vi "Launcher.vi"() -> ()   [LabVIEW 2022 SP3]
uses:
  Dynamic Load/Dynamic Load.lvclass
panel:
  in  "Dynamic Load.lvclass":refnum<class "Dynamic Load.lvclass">
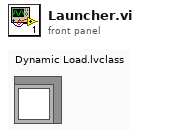
[diagram p1: front panel]
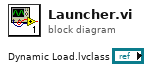
[diagram p0: block diagram]
diagram:
